vi "Get Heater Temp.vi"(8 "Ramb config":cluster{"Tamb":dbl, "Ramb":dbl}={"Tamb"=25.0, "Ramb"=10.0} {"Ramb" format="%.3f"; "Tamb" format="%.3f"}, 9 "TCR config":T2={"TCR1"=0.00205, "TCR2"=3e-07, "TRH"=0.766, "TRM"=0.928} {"TRM" format="%.3f"; "TRH" format="%.3f"; "TCR2" format="%.2e"; "TCR1" format="%.2e"}, 10 "Channel config":T3={"Voltage channel index"=0, "Current channel index"=1}, 11 "array":waveform(dbl)[](array[waveform])) -> (2 "Channel names":T1, 3 "waveform out":waveform(dbl))   [LabVIEW 2019]
doc: "This example demonstrates how to acquire a continuous amount of data (Waveform) using the DAQ device's internal clock. It also shows how to synchronize two devices for different device families (E Series, S Series, M Series, X Series, DSA, and SC Express), to simultaneously acquire the data.\n\nFor instructions on how to connect your signals to the DAQ device, refer to your device documentation."
panel:
  # "Get Heater Temperature"
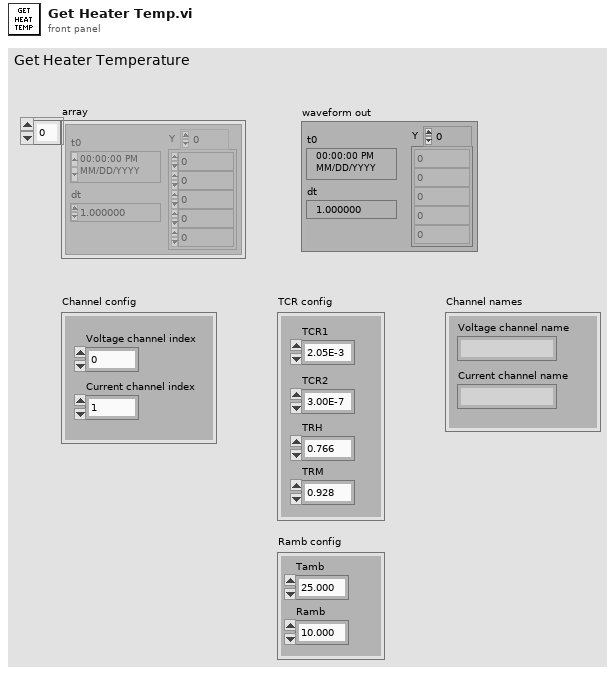
[diagram p1: front panel]
types:
  T1 = cluster{"Voltage channel name":string, "Current channel name":string}
  T2 = cluster{"TCR1":dbl, "TCR2":dbl, "TRH":dbl, "TRM":dbl}
  T3 = cluster{"Voltage channel index":i32, "Current channel index":i32}
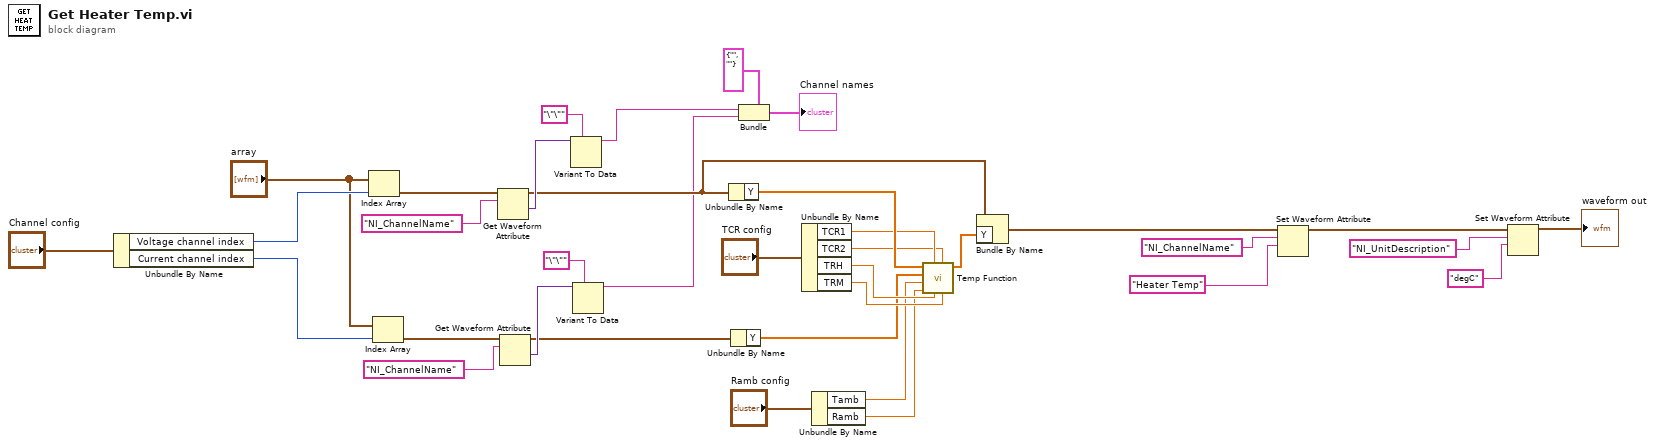
[diagram p0: block diagram]
diagram:
  n1 = Unbundle By Name("Channel config") -> ("Voltage channel index"=w28:i32, "Current channel index"=w20:i32)
  n2 = Index Array(array="array", index=w28) -> (element=w32:waveform(dbl))
  n3 = Index Array(array="array", index=w20) -> (element=w25:waveform(dbl))
  n4 = Get Waveform Attribute(6:"NI_ChannelName" ("name"), 7:w32) -> (1:w26:variant, 3:w8:waveform(dbl))  [unwired: 2 in, 2 out]
  n5 = Get Waveform Attribute(6:"NI_ChannelName" ("name"), 7:w25) -> (1:w23:variant, 3:w22:waveform(dbl))  [unwired: 2 in, 2 out]
  n6 = Variant To Data(type="\"\"" ("name"), Variant=w26) -> (data=w6:string)  [unwired: 1 in, 1 out]
  n7 = Variant To Data(type="\"\"" ("name"), Variant=w23) -> (data=w5:string)  [unwired: 1 in, 1 out]
  n8 = Unbundle By Name(w8) -> ("Y"=w18:dbl[])
  n9 = Unbundle By Name(w22) -> ("Y"=w1:dbl[])
  n10 = Bundle(cluster=cluster{"name":string, "name 2":string} {"name"="", "name 2"=""} ("input cluster"), "name"=w6, "name 2"=w5) -> (→"Channel names":cluster{"name":string, "name 2":string})
  n11 = Unbundle By Name("TCR config") -> ("TCR1"=w16:dbl, "TCR2"=w15:dbl, "TRH"=w14:dbl, "TRM"=w13:dbl)
  n12 = Unbundle By Name("Ramb config") -> ("Tamb"=w11:dbl, "Ramb"=w10:dbl)
  n13 = call "Temp Function.vi"("TRM"=w13, "TCR2"=w15, "TRH"=w14, "TCR1"=w16, "Ramb"=w10, "Tamb"=w11, "I"=w1, "V"=w18) -> ("Tamb"=w9:dbl[])  [unwired: 3 in]
  n14 = Bundle By Name(cluster=w8, "Y"=w9) -> (w7:waveform(dbl))
  n15 = Set Waveform Attribute(5:"Heater Temp" ("name"), 6:"NI_ChannelName" ("name"), 7:w7) -> (3:w34:waveform(dbl))  [unwired: 1 in, 2 out]
  n16 = Set Waveform Attribute(5:"degC" ("name"), 6:"NI_UnitDescription" ("name"), 7:w34) -> (3:→"waveform out":waveform(dbl))  [unwired: 1 in, 2 out]
